vi "Get Repo Path.vi"(8 "error in (no error)":errorcluster, 11 "VI / lvlib / class / Folder Path":path) -> (0 "error out":errorcluster, 2 "Repo Exist?":bool, 3 "Repo Path":path)   [LabVIEW 2019, in "Hawkeye.lvlib"]
uses:
  Hawkeye.lvlib
  <userlib>/_OpenG.lib/file/file.llb/File Exists - Scalar__ogtk.vi
  <userlib>/_OpenG.lib/file/file.llb/Valid Path - Traditional__ogtk.vi
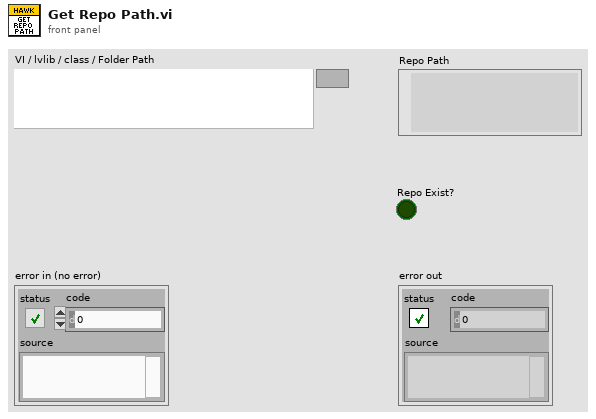
[diagram p1: front panel]
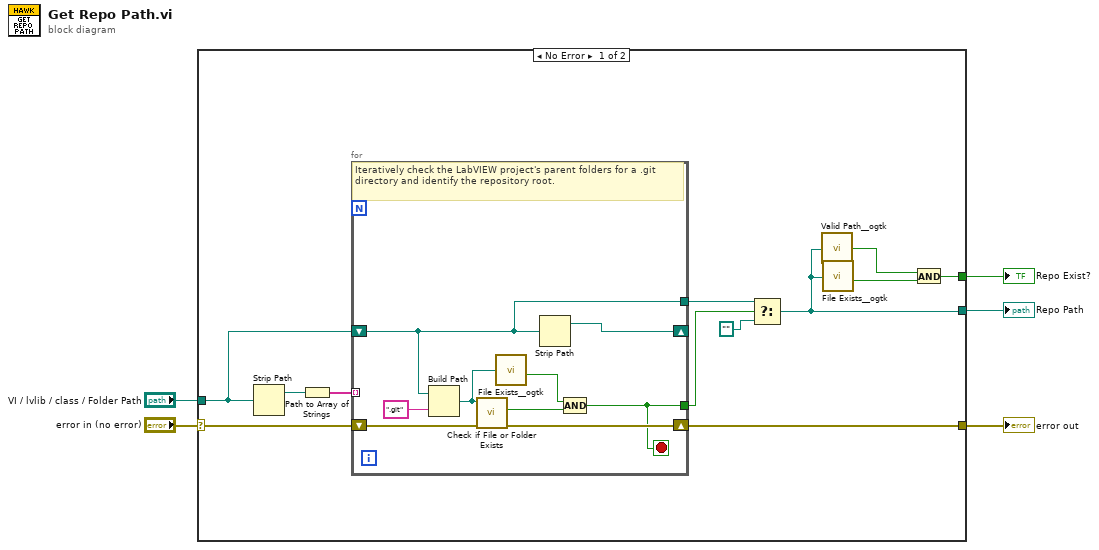
[diagram p0: block diagram]
diagram:
  n1 = case shown="No Error" "error in (no error)" {
    selector: "error in (no error)" -> [w13 w27]
    tunnel: [w7 _] -> w5
    tunnel: [w14 w27] -> w4
    tunnel: "VI / lvlib / class / Folder Path" -> [w10 _]
    tunnel: [w6 _] -> w1
    frame No Error {
      n2 = Strip Path(path=w10) -> (stripped path=w11:path)  [unwired: 1 out]
      n3 = Path to Array of Strings(0:w11) -> (2:w12:string[])  [unwired: 1 out]
      n4 = for {
        tunnel: w12 -> [_] mode=indexing
        shift-right: [w21] -> _
        shift-left: w10 -> [w22]
        tunnel: [w22] -> w16
        tunnel: [w19] -> w17
        shift-right: [w23] -> w14
        shift-left: w13 -> [w24]
        stop <- w19 stop-if-true
        # "Iteratively check the LabVIEW project's parent folders for a .git directory and identify the repository root."
        n5 = Build Path(base path=w22, name or relative path=".git") -> (appended path=w20:path)
        n6 = call <vilib>:"Check if File or Folder Exists.vi"("error in (no error)"=w24, "path"=w20) -> ("error out"=w23:errorcluster, "file or folder exists?"=w25:bool)  [unwired: 7 in, 1 out]
        n7 = call-poly <userlib>:"File Exists__ogtk.vi"("file path"=w20) -> ("exists"=w18:bool)  [unwired: 6 in, 1 out]
        n8 = Strip Path(path=w22) -> (stripped path=w21:path)  [unwired: 1 out]
        n9 = Compound Arithmetic op=AND(w18, w25) -> (w19:bool)
      }
      n10 = Select(t=w16, s=w17, f=path "") -> (s? t:f=w7:path)
      n11 = call-poly <userlib>:"Valid Path__ogtk.vi"("path"=w7) -> ("valid"=w8:bool)
      n12 = call-poly <userlib>:"File Exists__ogtk.vi"("file path"=w7) -> ("exists"=w9:bool)  [unwired: 6 in, 1 out]
      n13 = And(x=w8, y=w9) -> (x .and. y?=w6:bool)
    }
    frame Error {
    }
  }
  "Repo Path" <- w5
  "error out" <- w4
  "Repo Exist?" <- w1
